vi "Connect to IP Address.vi"(8 "error in (no error)":errorcluster, 11 "Device Ref in":T1 format="%.0x") -> (0 "error out":errorcluster, 2 "REST Client out":refnum<class "REST Client.lvclass">, 3 "Item Ref out":T1 format="%.0x")   [LabVIEW 2021, in "G5 Regatron Custom Device Engine.lvlib"]
uses:
  G5 Regatron Custom Device Engine.lvlib
  G5 LabVIEW REST API/Regatron.G5.Rest.lvlib
  <vilib>/NI VeriStand/Custom Device API/Custom Device API.lvlib
  <vilib>/NI VeriStand/Custom Device API/Get Item Property (String).vi
  Shared/Constants.vi
  Shared/G5 Regatron Custom Device Shared.lvlib
  <vilib>/NI VeriStand/Custom Device API/Custom Device Item Ref.ctl
  <vilib>/Addons/_JKI.lib/REST Client/classes/REST Client/REST Client.lvclass
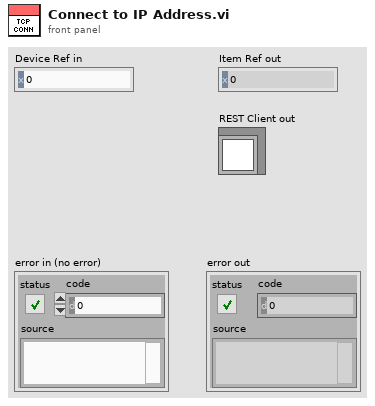
[diagram p1: front panel]
types:
  T1 = typedef "Custom Device API.lvlib/Custom Device Item Ref.ctl" = u64
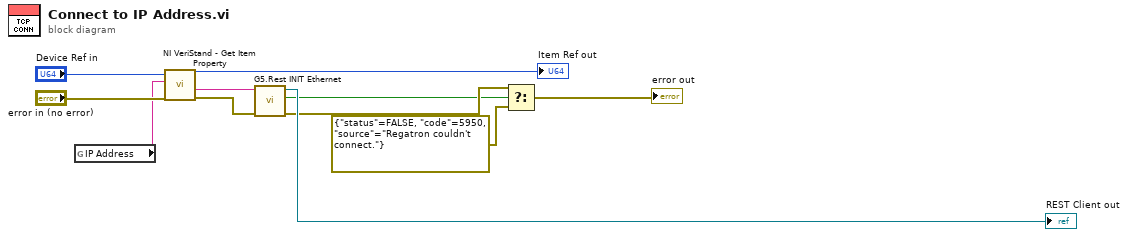
[diagram p0: block diagram]
diagram:
  n1 = global read "Constants.vi" "IP Address"() -> (w1:string)
  n2 = call-poly <vilib>:"NI VeriStand - Get Item Property.vi"("error in (no error)"="error in (no error)", "Property Name"=w1, "Item Ref in"="Device Ref in") -> ("error out"=w3:errorcluster, "Value"=w2:string, "Item Ref out"=→"Item Ref out":T1)  [unwired: 5 in, 1 out]
  n3 = call "G5.Rest INIT Ethernet.vi"("error in (no error)"=w3, "IP"=w2) -> ("error out"=w5:errorcluster, "Device found"=w4:bool, "G5 WEB API"=→"REST Client out":refnum<class "REST Client.lvclass">)  [unwired: 5 in, 2 out]
  n4 = Select(t=w5, s=w4, f=errorcluster {"status"=FALSE, "code"=5950, "source"="Regatron couldn't connect."}) -> (s? t:f=→"error out":errorcluster)
